vi "Start Drag Operation.vi"(8 "error in (no error)":errorcluster, 10 "Coords":T1, 11 "Table in":refnum<vi>) -> (0 "error out":errorcluster)   [LabVIEW 2016, in "UserInterface.lvlib" / "UserInterface.lvclass"]
uses:
  UserInterface.lvclass
  <vilib>/Utility/miscctls.llb/LVPoint32TypeDef.ctl
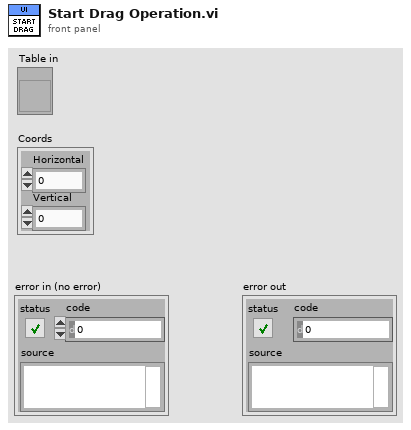
[diagram p1: front panel]
types:
  T1 = typedef "LVPoint32TypeDef.ctl" = cluster{"Horizontal":i32, "Vertical":i32}
  T2 = typedef "LVRowAndColumnTypeDef.ctl" = cluster{"Row":i32, "Column":i32}
  T3 = cluster{"data name":string, "drag data":variant}[]
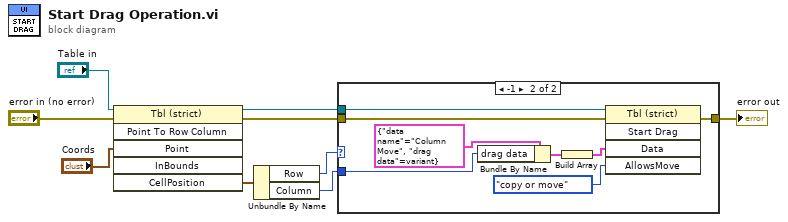
[diagram p0: block diagram]
diagram:
  n1 = invoke on="Invoke Node" class="Tbl (strict)" method="Point To Row Column"(reference="Table in", error in="error in (no error)", "Point"="Coords") -> (reference out=w4:refnum<vi>, error out=w2:errorcluster, "CellPosition"=w9:T2)  [unwired: 3 in, 3 out]
  n2 = Unbundle By Name(w9) -> ("Row"=w6:i32, "Column"=w5:i32)
  n3 = case shown="-1" w6 {
    tunnel: w5 -> [_ w16]
    tunnel: w4 -> [_ w13]
    tunnel: w2 -> [w10 w12]
    tunnel: [w10 w11] -> w1
    frame Default {
    }
    frame -1 {
      n4 = Bundle By Name(cluster=cluster{"data name":string, "drag data":variant} {"data name"="Column Move", "drag data"=variant}, "drag data"=w16) -> (w15:cluster{"data name":string, "drag data":variant})
      n5 = Build Array(w15) -> (w14:T3)
      n6 = invoke on="Invoke Node" class="Tbl (strict)" method="Start Drag"(reference=w13, error in=w12, "Data"=w14, "AllowsMove"=enum32{"copy or move", "copy only", "move only"}."copy or move" ("Drag Mode")) -> (error out=w11:errorcluster)  [unwired: 1 in, 4 out]
    }
  }
  "error out" <- w1
